vi "Generate Stub Service.vi"(8 "error in (no error)":errorcluster, 9 "gRPC Method Parameters in":T1[](array[typedef]), 10 ">>Application instance>>":refnum<vi>, 11 "Library in":refnum<vi>) -> (0 "error out":errorcluster, 1 "gRPC Method Parameters out":T1[](array[typedef]), 2 "LVClassLibrary out":refnum<vi>, 3 "Library out":refnum<vi>, 4 ">>Application instance>> out":refnum<vi>)   [LabVIEW 2019, in "gRPC Template Creation Utility.lvlib"]
uses:
  gRPC Template Creation Utility.lvlib
  TypeDefs/RPC Method Parameters.ctl
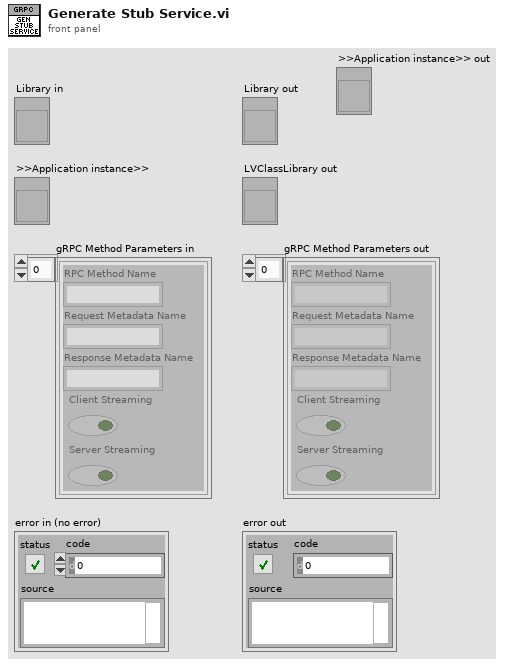
[diagram p1: front panel]
types:
  T1 = typedef "gRPC Template Creation Utility.lvlib/RPC Method Parameters.ctl" = cluster{"RPC Method Name":string, "Request Metadata Name":string, "Response Metadata Name":string, "Client Streaming":bool, "Server Streaming":bool}
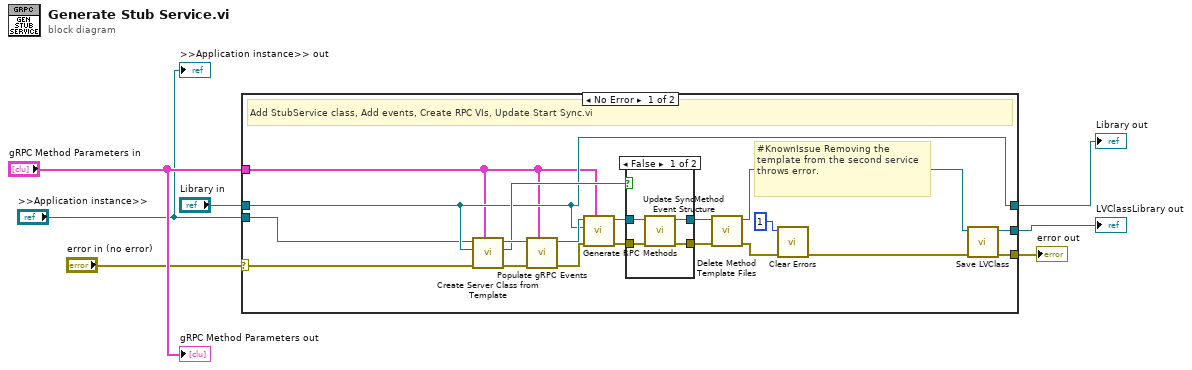
[diagram p0: block diagram]
diagram:
  n1 = case shown="No Error" "error in (no error)" {
    selector: "error in (no error)" -> [w11 w34]
    tunnel: [w26 w34] -> w7
    tunnel: [w25 _] -> w6
    tunnel: "gRPC Method Parameters in" -> [w9 _]
    tunnel: "Library in" -> [w10 w33]
    tunnel: ">>Application instance>>" -> [w8 _]
    tunnel: [w10 w33] -> w2
    frame No Error {
      # "#KnownIssue Removing the template from the second service throws error."
      # "Add StubService class, Add events, Create RPC VIs, Update Start Sync.vi"
      n2 = call "Create Server Class from Template.vi"("gRPC Method Parameters"=w9, "error in (no error)"=w11, "Library"=w10, "Application ref in"=w8) -> ("error out"=w12:errorcluster, "Already Exists ?"=w13:bool, "LVClassLibrary in"=w14:refnum<vi>)  [unwired: 5 in]
      n3 = call "Populate gRPC Events.vi"("RPC Method Parameters"=w9, "error in (no error)"=w12, "Server class in"=w14) -> ("error out"=w16:errorcluster, "Server class out"=w15:refnum<vi>)  [unwired: 7 in]
      n4 = call "Generate RPC Methods.vi"("RPC Method Parameters"=w9, "error in (no error)"=w16, "Library"=w10, "Server class in"=w15) -> ("error out"=w19:errorcluster, "Server class out"=w17:refnum<vi>)  [unwired: 6 in]
      n5 = case shown="False" w13 {
        tunnel: w17 -> [w30 w32]
        tunnel: [w29 w32] -> w18
        tunnel: w19 -> [w28 w31]
        tunnel: [w27 w31] -> w20
        frame False {
          n6 = call "Update SyncMethod Event Structure.vi"("error in (no error)"=w28, "Server class in"=w30) -> ("error out"=w27:errorcluster, "Server class out"=w29:refnum<vi>)  [unwired: 8 in]
        }
        frame True {
        }
      }
      n7 = call "Delete Method Template Files.vi"("error in (no error)"=w20, "LVClassLibrary in"=w18) -> ("error out"=w22:errorcluster, "LVClassLibrary out"=w24:refnum<vi>)  [unwired: 8 in]
      n8 = call <vilib>:"Clear Errors.vi"("error in (no error)"=w22, "specific error code to clear (0: all)"=1) -> ("error out"=w23:errorcluster)  [unwired: 4 in, 1 out]
      n9 = call "Save LVClass.vi"("error in (no error)"=w23, "LVClassLibrary in"=w24) -> ("error out"=w26:errorcluster, "LVClassLibrary out"=w25:refnum<vi>)  [unwired: 8 in]
    }
    frame Error {
    }
  }
  "Library out" <- w2
  "error out" <- w7
  "LVClassLibrary out" <- w6
  "gRPC Method Parameters out" <- "gRPC Method Parameters in"
  ">>Application instance>> out" <- ">>Application instance>>"
